vi "Sonar Sweep.vi"(11 "Input":string) -> (3 "# of increases":i32)   [LabVIEW 2020]
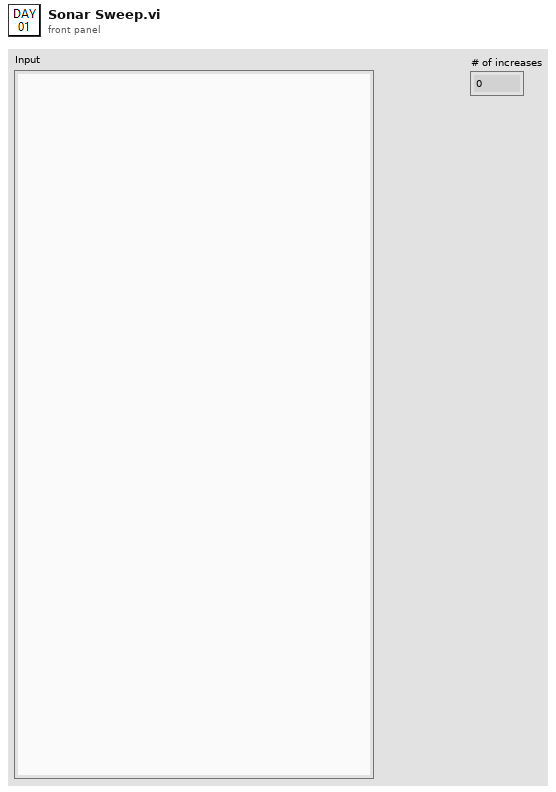
[diagram p1: front panel]
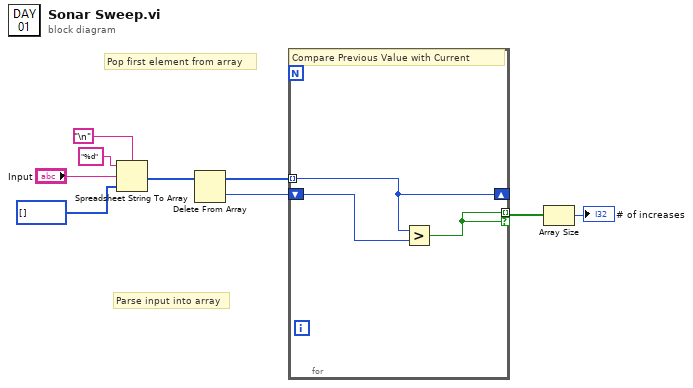
[diagram p0: block diagram]
diagram:
  # "Parse input into array"
  # "Pop first element from array"
  n1 = Spreadsheet String To Array(delimiter (Tab)="\n", format string="%d", spreadsheet string="Input", array type (2D Dbl)=i32[] []) -> (array=w5:i32[])
  n2 = Delete From Array(array=w5) -> (deleted portion=w3:i32, array with subset deleted=w4:i32[])  [unwired: 2 in]
  n3 = for {
    tunnel: w4 -> [w11] mode=indexing
    shift-right: [w11] -> _
    shift-left: w3 -> [w12]
    tunnel: [w10] -> w2 mode=indexing if=w10
    # "Compare Previous Value with Current"
    n4 = Greater?(x=w11, y=w12) -> (0:w10:bool)
  }
  n5 = Array Size(array=w2) -> (size(s)=→"# of increases":i32)
